vi "Create JSON Cluster.vi"(0 "Front Panel Ref In":refnum<vi>, 5 "JSON String":string, 11 "Error In":errorcluster) -> (4 "Parent Ref Out":refnum<vi>[](array[refnum]), 15 "Error Out":errorcluster)   [LabVIEW 2019, in "SLL JSON to Cluster.lvlib"]
doc: "This VI starts creating equivakent cluster from JSON tokens"
uses:
  SLL JSON to Cluster.lvlib
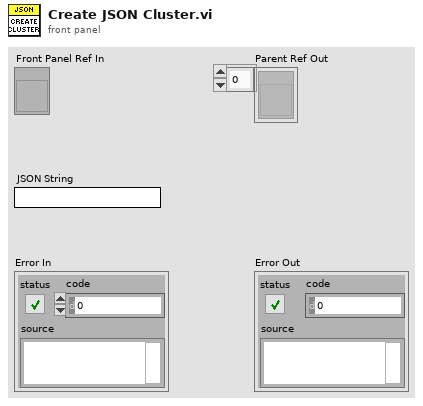
[diagram p1: front panel]
types:
  T1 = typedef "SLL JSON to Cluster.lvlib/Tokens.ctl" = enum16{"End", "Boolean", "Named Cluster", "Unnamed Cluster", "Array", "String", "Decimal", "FloatingPoint", "End Array", "End Cluster"}
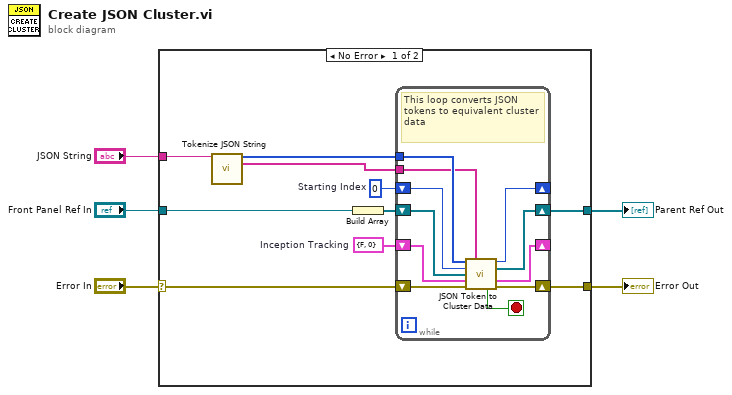
[diagram p0: block diagram]
diagram:
  n1 = case shown="No Error" "Error In" {
    selector: "Error In" -> [w11 w27]
    tunnel: [w15 _] -> w5
    tunnel: "JSON String" -> [w14 _]
    tunnel: [w13 w27] -> w3
    tunnel: "Front Panel Ref In" -> [w12 _]
    frame No Error {
      w7 = cluster{"In Array?":bool, "Cluster Level":i32} {"In Array?"=FALSE, "Cluster Level"=0}  # Inception Tracking
      w6 = 0  # Starting Index
      n2 = call "Tokenize JSON String.vi"("JSON String"=w14) -> ("Datatype Tokens"=w10:T1[], "Variable Names"=w9:string[])  [unwired: 12 in, 1 out]
      n3 = Build Array(w12) -> (w8:refnum<vi>[])
      n4 = while {
        tunnel: w10 -> [w24]
        tunnel: w9 -> [w23]
        shift-right: [w21] -> _
        shift-left: w6 -> [w22]
        shift-right: [w20] -> w15
        shift-left: w8 -> [w18]
        shift-right: [w19] -> _
        shift-left: w7 -> [w17]
        shift-right: [w25] -> w13
        shift-left: w11 -> [w26]
        stop <- w16 stop-if-true
        # "This loop converts JSON tokens to equivalent cluster data"
        n5 = call "JSON Token to Cluster Data.vi"("Token Array"=w24, "Variable Names"=w23, "Index"=w22, "Parent Ref In"=w18, "Inception Tracking In"=w17, "Error In"=w26) -> ("index out"=w21:i32, "Parent Ref Out"=w20:refnum<vi>[], "Inception Tracking Out"=w19:cluster{"In Array?":bool, "Cluster Level":i32}, "End?"=w16:bool, "Error Out"=w25:errorcluster)  [unwired: 5 in]
      }
    }
    frame Error {
    }
  }
  "Parent Ref Out" <- w5
  "Error Out" <- w3
